vi "AlazarSetExternalTrigger.vi"(3 "error in (no error)":errorcluster, 4 "Range":u32(ring)=2 items=["2.5V"=3, "5 V"=0, "1 V"=1, "TTL"=2], 5 "Coupling":u32(ring)=2 items=["AC"=1, "DC"=2], 6 "Handle":u32) -> (0 "error out":errorcluster, 1 "Return Code":u32, 2 "Handle":u32)   [LabVIEW 2021]
doc: "Set the external trigger range and coupling."
uses:
  ATSApi.dll
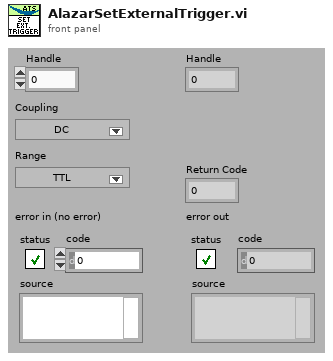
[diagram p1: front panel]
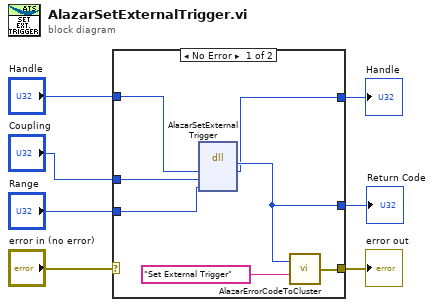
[diagram p0: block diagram]
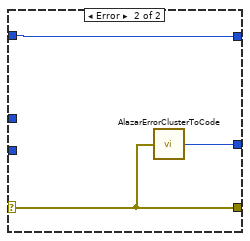
[diagram p2: hidden frame]
diagram:
  n1 = case shown="No Error" "error in (no error)" {
    selector: "error in (no error)" -> [_ w17]
    tunnel: [w11 w17] -> w6
    tunnel: [w13 w16] -> w5
    tunnel: "Handle" -> [w14 w15]
    tunnel: [w10 w15] -> w4
    tunnel: "Coupling" -> [w9 _]
    tunnel: "Range" -> [w8 _]
    frame No Error {
      n2 = dll-call lib="ATSApi.dll" fn="AlazarSetExternalTrigger"("handle"=w14, "coupling"=w9, "range"=w8) -> (w13:u32, "handle"=w10:u32)  [unwired: 5 in, 2 out]
      n3 = call "AlazarErrorCodeToCluster.vi"("Message"="Set External Trigger", "Error Code"=w13) -> ("error out"=w11:errorcluster)
    }
    frame Error {
      n4 = call "AlazarErrorClusterToCode.vi"("error in (no error)"=w17) -> ("Error Code"=w16:u32)
    }
  }
  "Handle" <- w4
  "error out" <- w6
  "Return Code" <- w5
